vi "Write lfData.vi"(8 "error in":errorcluster, 10 "LF Task":refnum<k21>, 11 "CRDS Data in":refnum<class "CRDS Data.lvclass">) -> (0 "error out":errorcluster, 3 "CRDS Data out":refnum<class "CRDS Data.lvclass">)   [LabVIEW 2011]
doc: "Retrieve the housekeeping data from the M-series card. Get all of the data that is available (don't wait for any specific amount). Take the mean of the data avaliable as the current 1 Hz value and then stuff the values into the appropriate cell values."
uses:
  CRDS Data.lvclass
  PAS_CRDS new/CRDS/Controls/lf_meas_type.ctl
  <vilib>/DAQmx/read.llb/DAQmx Read (Analog 2D DBL NChan NSamp).vi
  <vilib>/DAQmx/miscellaneous.llb/DAQmx Fill In Error Info.vi
  <vilib>/Analysis/NI_AALBase.lvlib
  Program Files/National Instruments/LabVIEW 2011/resource/objmgr/daqmx.rc
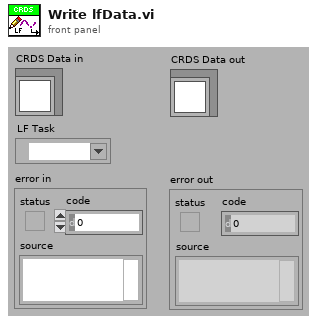
[diagram p1: front panel]
types:
  T1 = typedef "lf_meas_type.ctl" = enum16{"Trh", "P", "RHw", "T1"}
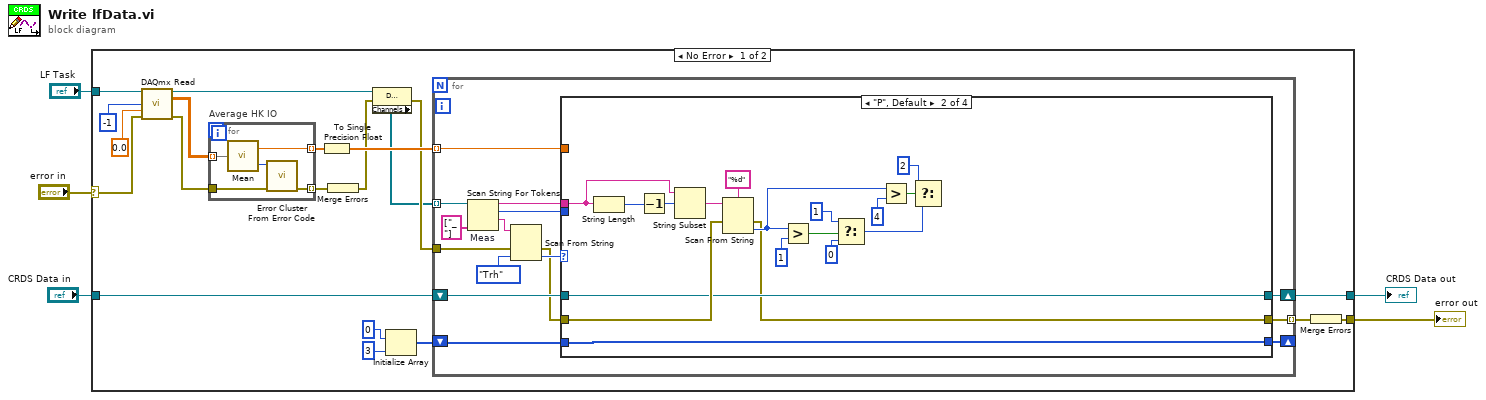
[diagram p0: block diagram]
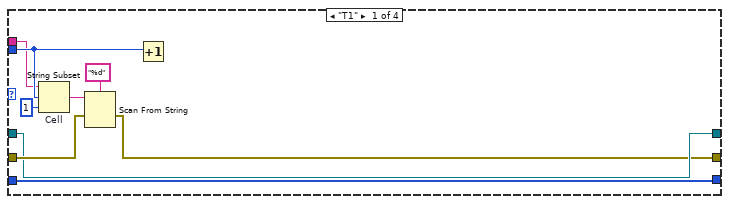
[diagram p2: hidden frame]
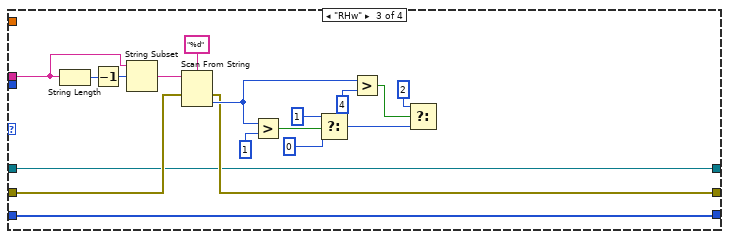
[diagram p3: hidden frame]
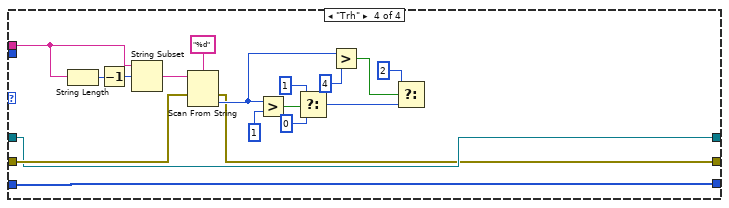
[diagram p4: hidden frame]
diagram:
  n1 = case shown="No Error" "error in" {
    selector: "error in" -> [w20 w110]
    tunnel: [w7 w110] -> w4
    tunnel: [w13 w109] -> w2
    tunnel: "CRDS Data in" -> [w18 w109]
    tunnel: "LF Task" -> [w19 _]
    frame No Error {
      n2 = call-poly <vilib>:"DAQmx Read.vi"("task/channels in"=w19, "number of samples per channel"=-1, "timeout"=0.0, "error in"=w20) -> ("task out"=w21:refnum<k21>, "data"=w23:dbl[][], "error out"=w10:errorcluster)  [unwired: 9 in]
      n3 = for "Average HK IO" {
        tunnel: w23 -> [w108] mode=indexing
        tunnel: [w107] -> w22 mode=indexing
        tunnel: w10 -> [w105]
        tunnel: [w104] -> w12 mode=indexing
        n4 = call <vilib>:"Mean.vi"("X"=w108) -> ("mean"=w107:dbl, "error"=w106:i32)
        n5 = call <vilib>:"Error Cluster From Error Code.vi"("error in (no error)"=w105, "error code (0)"=w106) -> ("error out"=w104:errorcluster)  [unwired: 7 in]
      }
      n6 = To Single Precision Float(number=w22) -> (single precision float=w17:sgl[])
      n7 = Merge Errors(w12) -> (w11:errorcluster)
      n8 = property class="DAQmx Task"(reference=w21, error in=w11) -> (error out=w9:errorcluster, "Channels"=w6:refnum<k21>[])  [unwired: 1 out]
      n9 = Initialize Array(0, 3 ("dimension size")) -> (w14:i32[])
      n10 = for {
        tunnel: w17 -> [w34] mode=indexing
        tunnel: w6 -> [w39] mode=indexing
        shift-right: [w32] -> _
        shift-left: w14 -> [w33]
        shift-right: [w31] -> w13
        shift-left: w18 -> [w40]
        tunnel: w9 -> [w30]
        tunnel: [w29] -> w8 mode=indexing
        n11 = Scan String For Tokens "Meas"(6:string[] ["_"] ("delimiters (\\s,\\t,\\r,\\n)"), 9:w39) -> (1:w36:string, 2:w26:i32, 3:w27:string)  [unwired: 4 in, 1 out]
        n12 = Scan From String(input string=w36, error in=w30, default 1=lf_meas_type."Trh" ("mType")) -> (error out=w28:errorcluster, output 1=w35:T1)  [unwired: 2 in, 2 out]
        n13 = case shown="\"P\", Default" w35 {
          tunnel: w40 -> [w42 w51 w68 w87]
          tunnel: w34 -> [_ _ _ _]
          tunnel: w33 -> [w49 w67 w72 w103]
          tunnel: [w49 w67 w72 w103] -> w32
          tunnel: [w42 w51 w68 w87] -> w31
          tunnel: w28 -> [w46 w52 w70 w88]
          tunnel: [w41 w50 w69 w86] -> w29
          tunnel: w27 -> [w43 w53 w71 w89]
          tunnel: w26 -> [w44 _ _ _]
          frame "T1" {
            n14 = String Subset "Cell"(string=w43, offset (0)=w44, length (rest)=1 ("length (rest)")) -> (substring=w47:string)
            n15 = Scan From String(format string="%d", input string=w47, error in=w46) -> (error out=w41:errorcluster)  [unwired: 3 in, 2 out]
            n16 = Increment(x=w44) -> ()  [unwired: 1 out]
          }
          frame "P", Default {
            n17 = String Length(string=w53) -> (length=w66:i32)
            n18 = Decrement(x=w66) -> (x-1=w65:i32)
            n19 = String Subset(string=w53, offset (0)=w65) -> (substring=w63:string)  [unwired: 1 in]
            n20 = Scan From String(format string="%d", input string=w63, error in=w52) -> (error out=w50:errorcluster, output 1=w58:i32)  [unwired: 2 in, 2 out]
            n21 = Greater?(x=w58, y=1) -> (0:w61:bool)
            n22 = Select(t=1 ("y"), s=w61, f=0) -> (s? t:f=w55:i32)
            n23 = Greater?(x=w58, y=4) -> (0:w56:bool)
            n24 = Select(t=2, s=w56, f=w55) -> ()  [unwired: 1 out]
          }
          frame "RHw" {
            n25 = String Length(string=w71) -> (length=w85:i32)
            n26 = Decrement(x=w85) -> (x-1=w84:i32)
            n27 = String Subset(string=w71, offset (0)=w84) -> (substring=w82:string)  [unwired: 1 in]
            n28 = Scan From String(format string="%d", input string=w82, error in=w70) -> (error out=w69:errorcluster, output 1=w77:i32)  [unwired: 2 in, 2 out]
            n29 = Greater?(x=w77, y=1) -> (0:w80:bool)
            n30 = Select(t=1 ("y"), s=w80, f=0) -> (s? t:f=w74:i32)
            n31 = Greater?(x=w77, y=4) -> (0:w75:bool)
            n32 = Select(t=2, s=w75, f=w74) -> ()  [unwired: 1 out]
          }
          frame "Trh" {
            n33 = String Length(string=w89) -> (length=w102:i32)
            n34 = Decrement(x=w102) -> (x-1=w101:i32)
            n35 = String Subset(string=w89, offset (0)=w101) -> (substring=w99:string)  [unwired: 1 in]
            n36 = Scan From String(format string="%d", input string=w99, error in=w88) -> (error out=w86:errorcluster, output 1=w94:i32)  [unwired: 2 in, 2 out]
            n37 = Greater?(x=w94, y=1) -> (0:w97:bool)
            n38 = Select(t=1 ("y"), s=w97, f=0) -> (s? t:f=w91:i32)
            n39 = Greater?(x=w94, y=4) -> (0:w92:bool)
            n40 = Select(t=2, s=w92, f=w91) -> ()  [unwired: 1 out]
          }
        }
      }
      n41 = Merge Errors(w8) -> (w7:errorcluster)
    }
    frame Error {
    }
  }
  "error out" <- w4
  "CRDS Data out" <- w2
